vi "emi_In single screen.vi"(5 "VI Refnum(This vi)":refnum<vi>, 9 "error in (no error)":errorcluster) -> (6 "VI Refnum":refnum<vi>, 8 "Window in screen":bool, 10 "error out":errorcluster)   [LabVIEW 2011]
doc: "Describe...\n\n\nIf no VI ref in, then the VI containing this VI is used.\nIf VI has multiple panes, only the first pane will be used.\n\nOn error in: Does not run."
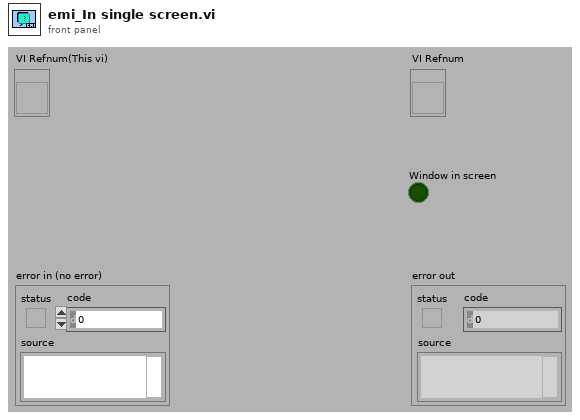
[diagram p1: front panel]
types:
  T1 = typedef "LVRectTypeDef.ctl" = cluster{"left":i16, "top":i16, "right":i16, "bottom":i16}
  T2 = typedef "LVAllMonitorsDisplayTypeDef.ctl" = cluster{"Bounds":cluster{"Left":i16, "Top":i16, "Right":i16, "Bottom":i16}, "Depth":i16}[]
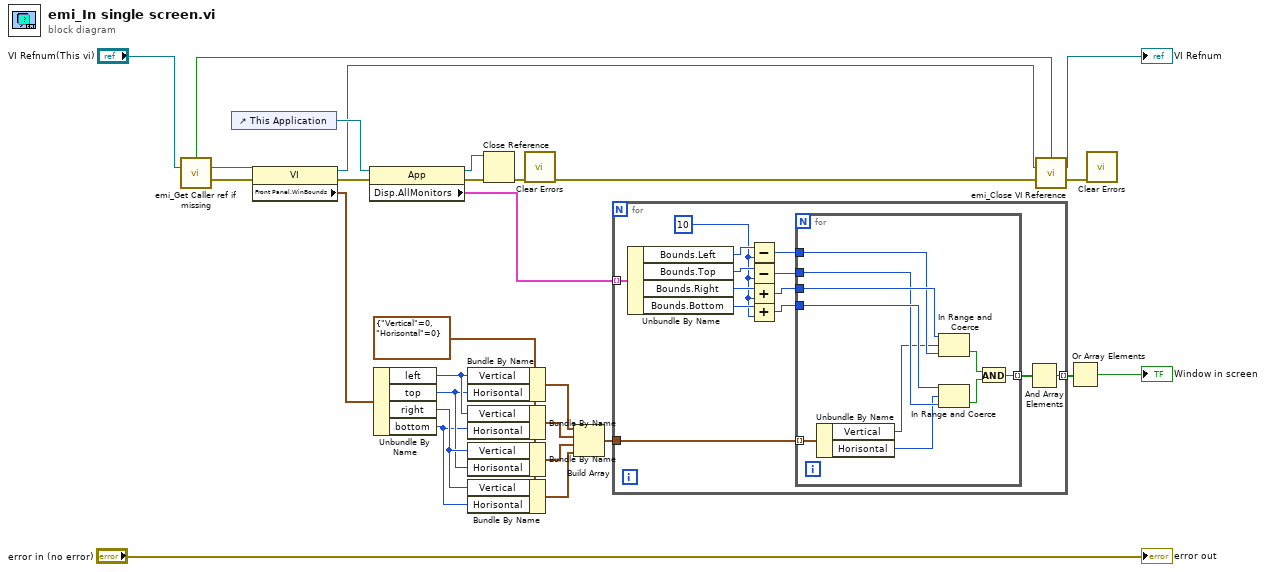
[diagram p0: block diagram]
diagram:
  w18 = cluster{"Vertical":i32, "Horisontal":i32} {"Vertical"=0, "Horisontal"=0}
  n1 = call "emi_Get Caller ref if missing.vi"("VI Refnum(Calling VI)"="VI Refnum(This vi)") -> ("Ref Generated"=w26:bool, "VI Refnum Out"=w4:refnum<vi>, "error out"=w5:errorcluster)  [unwired: 12 in]
  n2 = control-ref of="This Application"() -> (w11:refnum<vi>)
  n3 = property class="VI"(reference=w4, error in=w5) -> (reference out=w3:refnum<vi>, error out=w10:errorcluster, "Front Panel.WinBounds"=w25:T1)
  n4 = property class="App"(reference=w11, error in=w10) -> (reference out=w6:refnum<vi>, error out=w8:errorcluster, "Disp.AllMonitors"=w15:T2)
  n5 = Unbundle By Name(w25) -> ("left"=w24:i16, "top"=w22:i16, "right"=w23:i16, "bottom"=w21:i16)
  n6 = Bundle By Name(cluster=w18, "Vertical"=w24, "Horisontal"=w22) -> (w20:cluster{"Vertical":i32, "Horisontal":i32})
  n7 = Bundle By Name(cluster=w18, "Vertical"=w24, "Horisontal"=w21) -> (w19:cluster{"Vertical":i32, "Horisontal":i32})
  n8 = Bundle By Name(cluster=w18, "Vertical"=w23, "Horisontal"=w22) -> (w17:cluster{"Vertical":i32, "Horisontal":i32})
  n9 = Bundle By Name(cluster=w18, "Vertical"=w23, "Horisontal"=w21) -> (w16:cluster{"Vertical":i32, "Horisontal":i32})
  n10 = Close Reference(reference=w6, error in (no error)=w8) -> (error out=w7:errorcluster)
  n11 = call <vilib>:"Clear Errors.vi"("error in (no error)"=w7) -> ("error out"=w2:errorcluster)  [unwired: 6 in]
  n12 = Build Array(w20, w19, w17, w16) -> (w14:cluster{"Vertical":i32, "Horisontal":i32}[])
  n13 = for {
    tunnel: w15 -> [w41] mode=indexing
    tunnel: w14 -> [w40]
    tunnel: [w37] -> w13 mode=indexing
    w30 = i16 10 ("Bounds.Left")
    n14 = Unbundle By Name(w41) -> ("Bounds.Left"=w39:i16, "Bounds.Top"=w31:i16, "Bounds.Right"=w35:i16, "Bounds.Bottom"=w33:i16)
    n15 = Subtract(x=w39, y=w30) -> (x-y=w36:i16)
    n16 = Subtract(x=w31, y=w30) -> (x-y=w29:i16)
    n17 = Add(x=w35, y=w30) -> (x+y=w34:i16)
    n18 = Add(x=w33, y=w30) -> (x+y=w32:i16)
    n19 = for {
      tunnel: w40 -> [w47] mode=indexing
      tunnel: w32 -> [w49]
      tunnel: w34 -> [w51]
      tunnel: w29 -> [w48]
      tunnel: w36 -> [w50]
      tunnel: [w42] -> w38 mode=indexing
      n20 = Unbundle By Name(w47) -> ("Vertical"=w46:i32, "Horisontal"=w45:i32)
      n21 = In Range and Coerce(upper limit=w51, x=w46, lower limit=w50) -> (In Range?=w44:bool)  [unwired: 1 out]
      n22 = In Range and Coerce(upper limit=w49, x=w45, lower limit=w48) -> (In Range?=w43:bool)  [unwired: 1 out]
      n23 = And(x=w44, y=w43) -> (x .and. y?=w42:bool)
    }
    n24 = And Array Elements(Boolean array=w38) -> (logical AND=w37:bool)
  }
  n25 = call "emi_Close VI Reference.vi"("Close ref?(T)"=w26, "VI Refnum"=w3, "error in (no error)"=w2) -> ("VI Refnum Out"=→"VI Refnum":refnum<vi>, "error out"=w1:errorcluster)  [unwired: 11 in]
  n26 = Or Array Elements(Boolean array=w13) -> (logical OR=→"Window in screen":bool)
  n27 = call <vilib>:"Clear Errors.vi"("error in (no error)"=w1) -> ()  [unwired: 6 in, 1 out]
  "error out" <- "error in (no error)"
